vi "Cal Plot Scale.vi"(8 "error in (no error)":errorcluster, 11 "Domain_Steady_2D_Rect in":refnum<class "NI_Domain_Steady_2D_Rect.lvclass">) -> (0 "error out":errorcluster, 1 "Y Scale":T1, 2 "X Scale":T1, 3 "Domain_Steady_2D_Rect out":refnum<class "NI_Domain_Steady_2D_Rect.lvclass">, 4 "# of t-points":i32)   [LabVIEW 2017, in "NI_PDE.lvlib" / "NI_Domain_Steady_2D_Rect.lvclass"]
uses:
  <vilib>/gmath/pde.llb/DomainClass/Domain_Steady_2D_Rect/NI_Domain_Steady_2D_Rect.lvclass
  <vilib>/Utility/miscctls.llb/LVOffsetAndMultiplierTypeDef.ctl
  <vilib>/gmath/pde.llb/DomainClass/Domain_Steady_2D_Rect/NI_Domain_Steady_2D_Rect.lvclass/NI_Domain_Steady_2D_Rect.ctl
  <vilib>/gmath/NI_PDE.lvlib
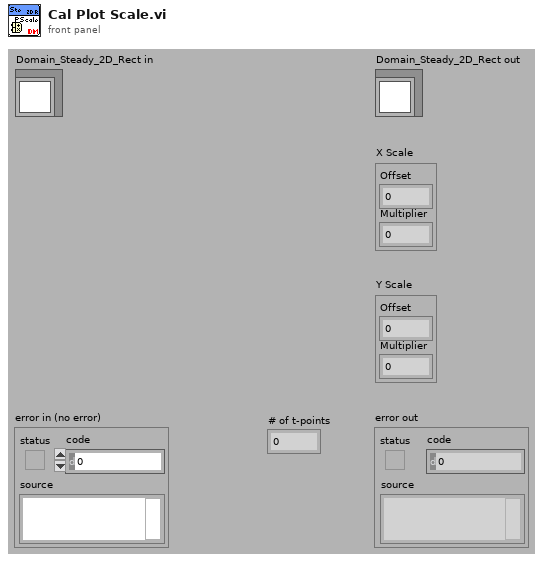
[diagram p1: front panel]
types:
  T1 = typedef "LVOffsetAndMultiplierTypeDef.ctl" = cluster{"Offset":dbl, "Multiplier":dbl}
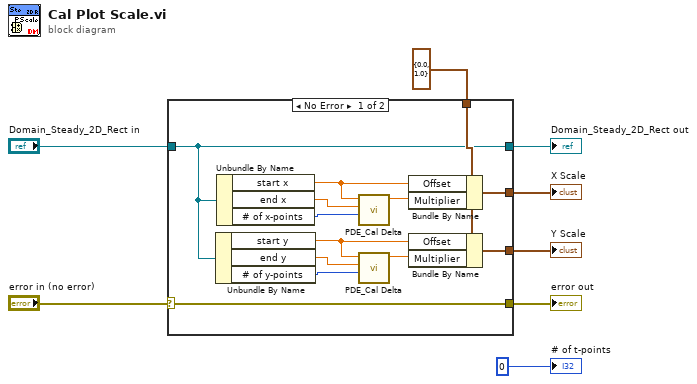
[diagram p0: block diagram]
diagram:
  n1 = case shown="No Error" "error in (no error)" {
    selector: "error in (no error)" -> [w9 w24]
    tunnel: "Domain_Steady_2D_Rect in" -> [w10 w23]
    tunnel: [w10 w23] -> w8
    tunnel: [w9 w24] -> w7
    tunnel: T1 {"Offset"=0.0, "Multiplier"=1.0} ("Offset and Multiplier") -> [w13 w22]
    tunnel: [w12 w22] -> w3
    tunnel: [w11 w22] -> w2
    frame No Error {
      n2 = Unbundle By Name(w10) -> ("start y"=w15:dbl, "end y"=w17:dbl, "# of y-points"=w16:i32)
      n3 = Unbundle By Name(w10) -> ("start x"=w20:dbl, "end x"=w18:dbl, "# of x-points"=w19:i32)
      n4 = call <vilib>:"PDE_Cal Delta.vi"("# of points"=w19, "end"=w18, "start"=w20) -> ("delta"=w21:dbl)  [unwired: 8 out]
      n5 = call <vilib>:"PDE_Cal Delta.vi"("# of points"=w16, "end"=w17, "start"=w15) -> ("delta"=w14:dbl)  [unwired: 8 out]
      n6 = Bundle By Name(cluster=w13, "Offset"=w20, "Multiplier"=w21) -> (w12:T1)
      n7 = Bundle By Name(cluster=w13, "Offset"=w15, "Multiplier"=w14) -> (w11:T1)
    }
    frame Error {
    }
  }
  "Domain_Steady_2D_Rect out" <- w8
  "error out" <- w7
  "X Scale" <- w3
  "Y Scale" <- w2
  "# of t-points" <- 0 ("# of t-points")
